vi "GAIN.vi"(0 "SR850 GPIB In":refnum<visa-resource-name>, 1 "Max. Hassasiyet":dbl=15.0, 2 "Auto Gain (False)":bool, 7 "Enum":enum16{"X", "Y"}(ring), 9 "Min. Hassasiyet":u16(ring) items=["100 nV", "200 nV", "500 nV", "1 uV", "2 uV", "5 uV", "10 uV", "20 uV", "50 uV", "100 uV", "200 uV", "500 uV", "1 mV"], 11 "error in":errorcluster, 13 "choose":dbl) -> (4 "SR850 GPIB Out":refnum<visa-resource-name>, 12 "y":dbl, 15 "error out":errorcluster)   [LabVIEW 2014]
uses:
  show_sensitivity.vi
panel:
  out "output":dbl
  out "abs(x)":dbl
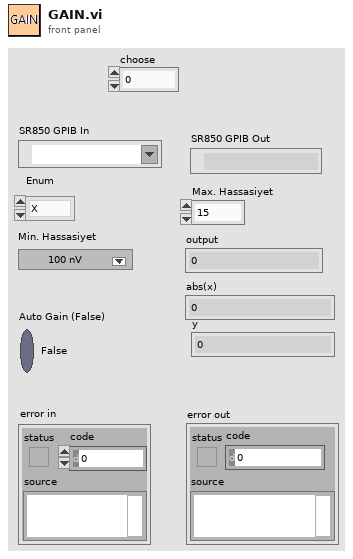
[diagram p1: front panel]
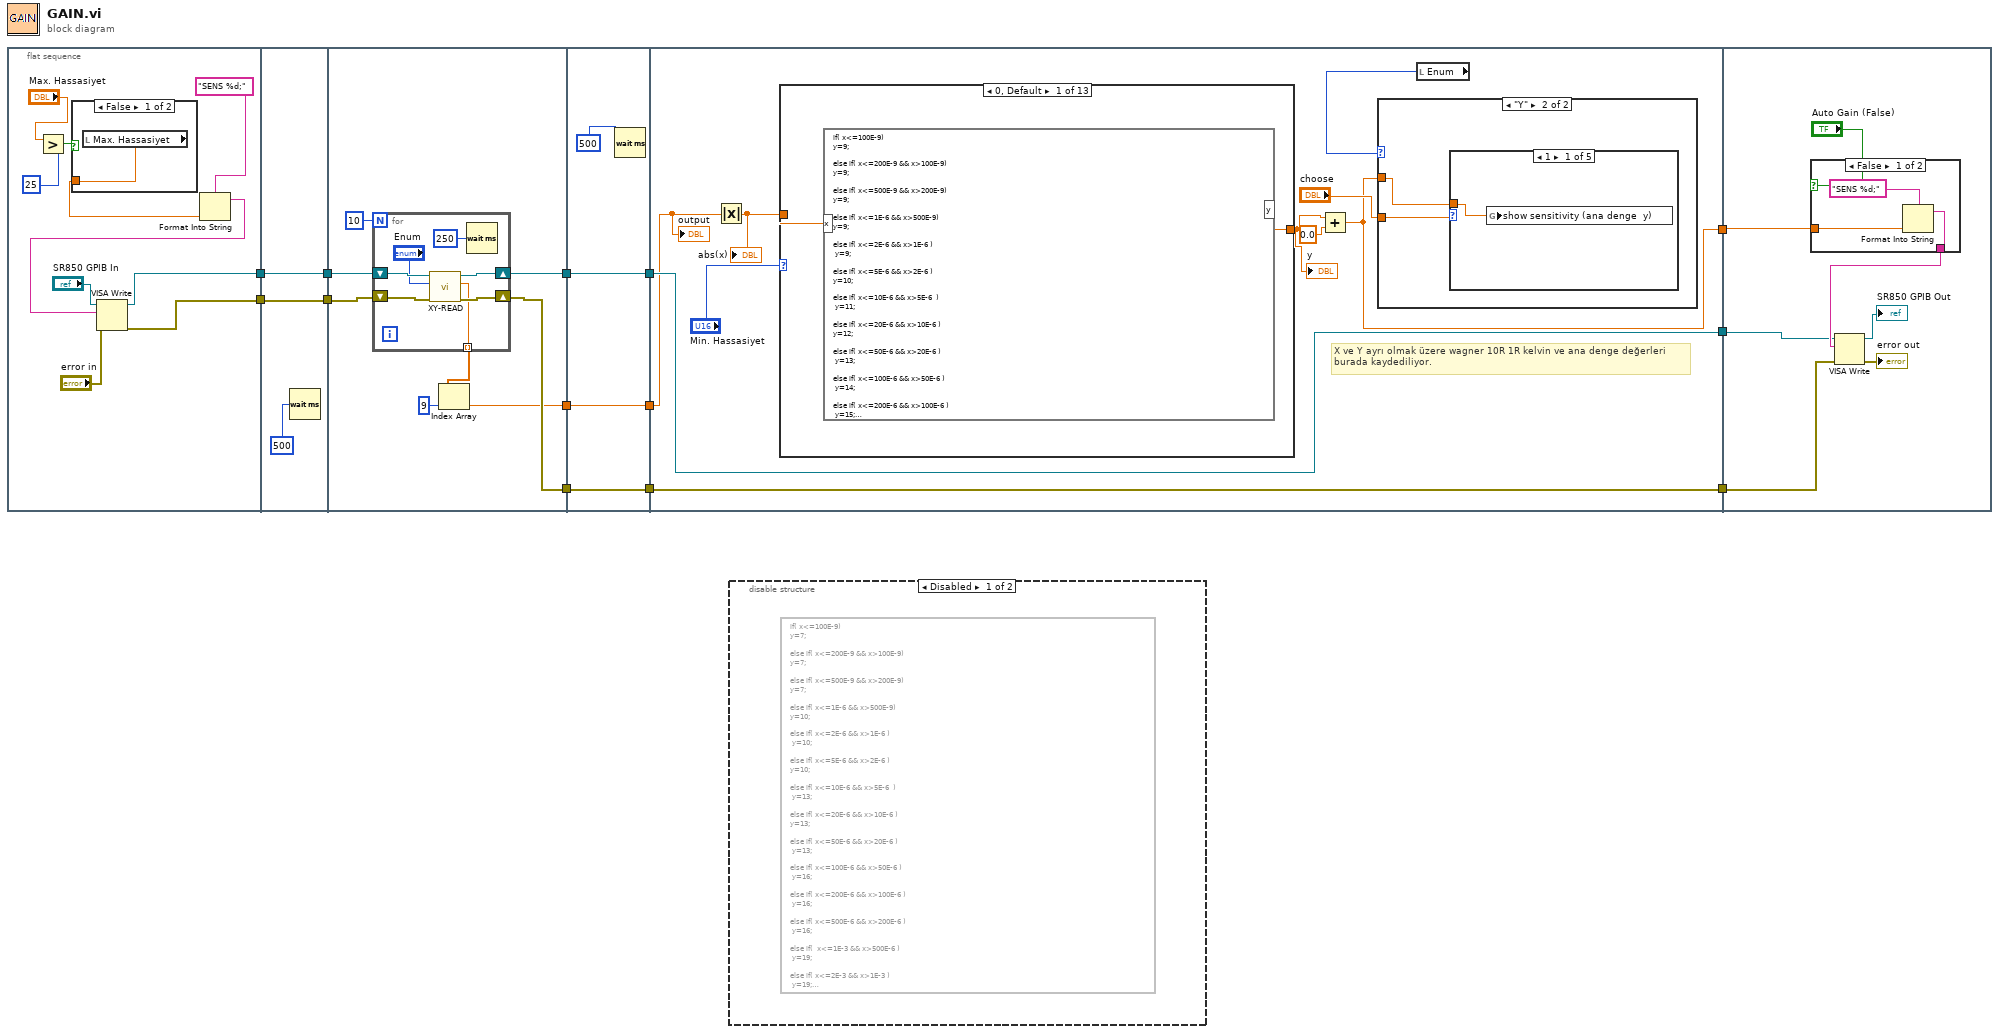
[diagram p0: block diagram]
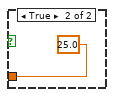
[diagram p3: hidden frame]
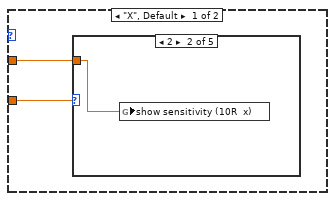
[diagram p4: hidden frame]
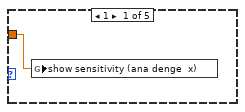
[diagram p5: hidden frame]
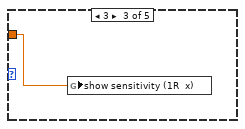
[diagram p6: hidden frame]
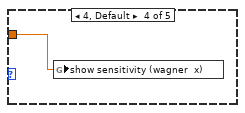
[diagram p7: hidden frame]
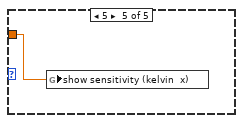
[diagram p8: hidden frame]
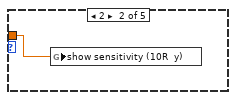
[diagram p9: hidden frame]
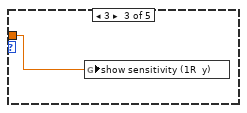
[diagram p10: hidden frame]
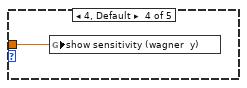
[diagram p11: hidden frame]
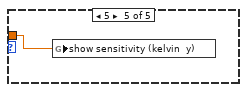
[diagram p12: hidden frame]
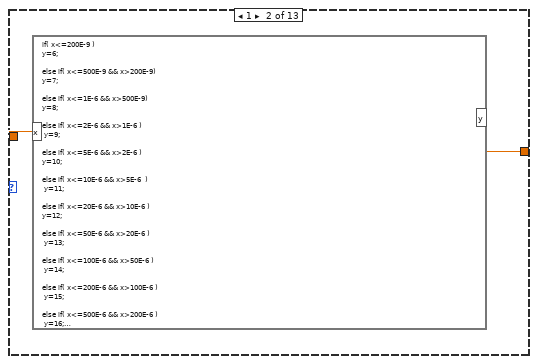
[diagram p13: hidden frame]
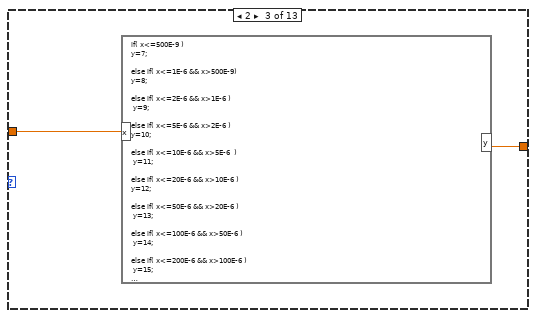
[diagram p14: hidden frame]
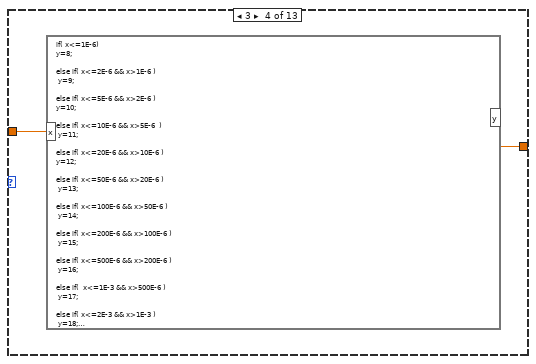
[diagram p15: hidden frame]
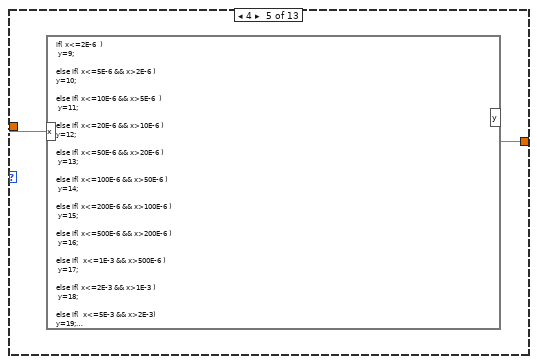
[diagram p16: hidden frame]
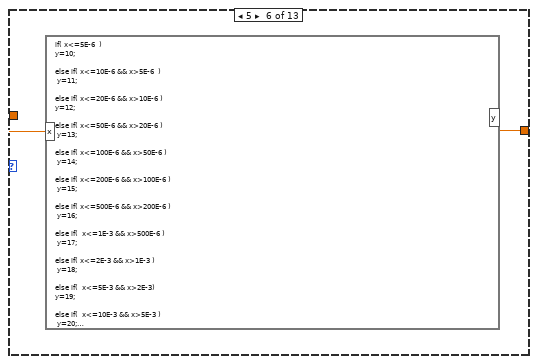
[diagram p17: hidden frame]
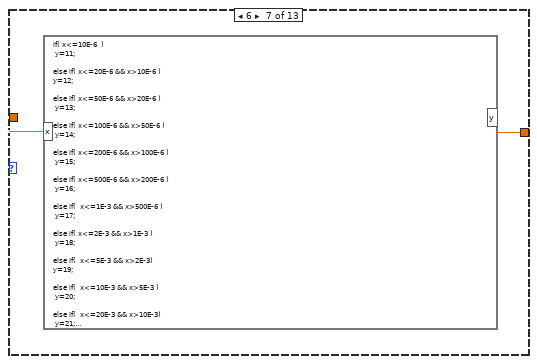
[diagram p18: hidden frame]
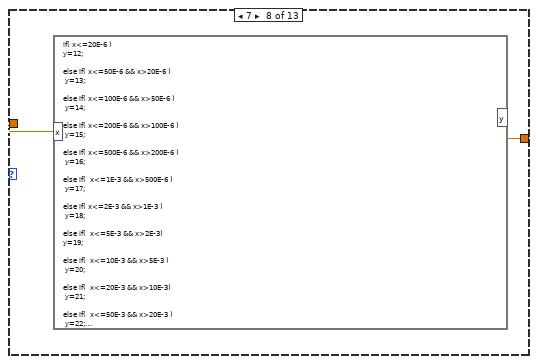
[diagram p19: hidden frame]
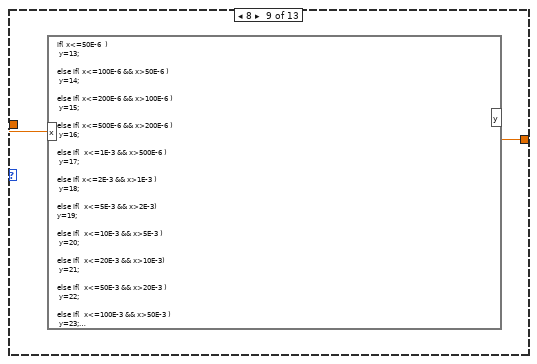
[diagram p20: hidden frame]
diagram:
  n1 = flat-sequence {
    tunnel: [w21] -> w10
    tunnel: [w18] -> w8
    tunnel: w10 -> [w28]
    tunnel: [w28] -> w9
    tunnel: w8 -> [w27]
    tunnel: [w27] -> w7
    tunnel: w9 -> [w36]
    tunnel: w7 -> [w35]
    tunnel: [w34] -> w6
    tunnel: [w33] -> w4
    tunnel: [w29] -> w2
    tunnel: w6 -> [w47]
    tunnel: [w47] -> w5
    tunnel: w4 -> [w46]
    tunnel: [w46] -> w3
    tunnel: w2 -> [w45]
    tunnel: [w45] -> w1
    tunnel: [w56] -> w13
    tunnel: w5 -> [w56]
    tunnel: [w55] -> w12
    tunnel: w3 -> [w55]
    tunnel: w1 -> [w53]
    tunnel: [w48] -> w11
    tunnel: w13 -> [w99]
    tunnel: w12 -> [w98]
    tunnel: w11 -> [w100]
    frame #0 {
      n2 = Greater?(x="Max. Hassasiyet", y=25) -> (0:w15:bool)
      n3 = case shown="False" w15 {
        tunnel: [w24 25.0] -> w14
        frame False {
          n4 = local read "Max. Hassasiyet"() -> (w24:dbl)
        }
        frame True {
        }
      }
      n5 = Format Into String(format string="SENS %d;", w14) -> (resulting string=w19:string)  [unwired: 2 in, 1 out]
      n6 = VISA Write(VISA resource name="SR850 GPIB In", write buffer=w19, error in (no error)="error in") -> (VISA resource name out=w21:refnum<visa-resource-name>, error out=w18:errorcluster)  [unwired: 1 out]
    }
    frame #1 {
      n7 = Wait (ms)(milliseconds to wait=u32 500) -> ()  [unwired: 1 out]
    }
    frame #2 {
      n8 = for {
        N: 10 -> [_]
        shift-right: [w41] -> w34
        shift-left: w36 -> [w43]
        shift-right: [w40] -> w33
        shift-left: w35 -> [w42]
        tunnel: [w38] -> w31 mode=indexing
        n9 = call "XY-READ.vi"("Error IN"=w42, "X/Y ?"="Enum", "SR850 GPIB IN"=w43) -> ("Error OUT"=w40:errorcluster, "SR850_Reading"=w38:dbl, "SR850 GPIB OUT"=w41:refnum<visa-resource-name>)  [unwired: 6 in]
        n10 = Wait (ms)(milliseconds to wait=u32 250) -> ()  [unwired: 1 out]
      }
      n11 = Index Array(array=w31, index=9) -> (element=w29:dbl)
    }
    frame #3 {
      n12 = Wait (ms)(milliseconds to wait=u32 500) -> ()  [unwired: 1 out]
    }
    frame #4 {
      # "X ve Y ayrı olmak üzere wagner 10R 1R kelvin ve ana denge değerleri\nburada kaydediliyor."
      n13 = Absolute Value(x=w53) -> (abs(x)=w54:dbl)
      "abs(x)" <- w54
      n14 = case shown="0, Default" "Min. Hassasiyet" {
        tunnel: [w73 w75 w76 w79 w81 w83 w84 w86 w88 w90 w92 w94 w96] -> w50
        tunnel: w54 -> [w72 w74 w77 w78 w80 w82 w85 w87 w89 w91 w93 w95 w97]
        frame 0, Default {
          n15 = formula code="if( x<=100E-9) \ny=9;\n\nelse if( x<=200E-9 && x>100E-9) \ny=9;\n\nelse if( x<=500E-9 && x>200E-9) \ny=9;\n\nelse if( x<=1E-6 && x>500E-9) \ny=9;\n\nelse if( x<=2E-6 && x>1E-6 ) \n\ty=9;\n\nelse if( x<=5E-6 && x>2E-6 ) \ny=10;\n\nelse if( x<=10E-6 && x>5E-6  ) \n\ty=11;\n\nelse if( x<=20E-6 && x>10E-6 ) \ny=12;\n\nelse if( x<=50E-6 && x>20E-6 ) \n\ty=13;\n\nelse if( x<=100E-6 && x>50E-6 ) \n\ty=14;\n\nelse if( x<=200E-6 && x>100E-6 ) \n\ty=15;\n\nelse if( x<=500E-6 && x>200E-6 ) \n\ty=16;\n\nelse if(  x<=1E-3 && x>500E-6 ) \n\ty=17;\n\nelse if( x<=2E-3 && x>1E-3 ) \n\ty=18;\n\nelse if(  x<=5E-3 && x>2E-3) \ny=19;\n\nelse if(  x<=10E-3 && x>5E-3 ) \n\ty=20;\n\nelse if(  x<=20E-3 && x>10E-3) \n\ty=21;\n\nelse if(  x<=50E-3 && x>20E-3 ) \n\ty=22;\n\nelse if(  x<=100E-3 && x>50E-3 ) \n\ty=23;\n\nelse if(  x<=200E-3 && x>100E-3 ) \n\ty=24;\n\nelse if(  x<=500E-3 && x>200E-3 ) \n\ty=25;\n\nelse if(  x<=1 && x>500E-3 ) \ny=26;\n\nelse \n\ty=26;"("x"=w72) -> ("y"=w73:dbl)
        }
        frame 1 {
          n16 = formula code="if( x<=200E-9 ) \ny=6;\n\nelse if( x<=500E-9 && x>200E-9) \ny=7;\n\nelse if( x<=1E-6 && x>500E-9) \ny=8;\n\nelse if( x<=2E-6 && x>1E-6 ) \n\ty=9;\n\nelse if( x<=5E-6 && x>2E-6 ) \ny=10;\n\nelse if( x<=10E-6 && x>5E-6  ) \n\ty=11;\n\nelse if( x<=20E-6 && x>10E-6 ) \ny=12;\n\nelse if( x<=50E-6 && x>20E-6 ) \n\ty=13;\n\nelse if( x<=100E-6 && x>50E-6 ) \n\ty=14;\n\nelse if( x<=200E-6 && x>100E-6 ) \n\ty=15;\n\nelse if( x<=500E-6 && x>200E-6 ) \n\ty=16;\n\nelse if(  x<=1E-3 && x>500E-6 ) \n\ty=17;\n\nelse if( x<=2E-3 && x>1E-3 ) \n\ty=18;\n\nelse if(  x<=5E-3 && x>2E-3) \ny=19;\n\nelse if(  x<=10E-3 && x>5E-3 ) \n\ty=20;\n\nelse if(  x<=20E-3 && x>10E-3) \n\ty=21;\n\nelse if(  x<=50E-3 && x>20E-3 ) \n\ty=22;\n\nelse if(  x<=100E-3 && x>50E-3 ) \n\ty=23;\n\nelse if(  x<=200E-3 && x>100E-3 ) \n\ty=24;\n\nelse if(  x<=500E-3 && x>200E-3 ) \n\ty=25;\n\nelse if(  x<=1 && x>500E-3 ) \ny=26;\n\nelse \n\ty=26;"("x"=w74) -> ("y"=w75:dbl)
        }
        frame 2 {
          n17 = formula code="if( x<=500E-9 ) \ny=7;\n\nelse if( x<=1E-6 && x>500E-9) \ny=8;\n\nelse if( x<=2E-6 && x>1E-6 ) \n\ty=9;\n\nelse if( x<=5E-6 && x>2E-6 ) \ny=10;\n\nelse if( x<=10E-6 && x>5E-6  ) \n\ty=11;\n\nelse if( x<=20E-6 && x>10E-6 ) \ny=12;\n\nelse if( x<=50E-6 && x>20E-6 ) \n\ty=13;\n\nelse if( x<=100E-6 && x>50E-6 ) \n\ty=14;\n\nelse if( x<=200E-6 && x>100E-6 ) \n\ty=15;\n\nelse if( x<=500E-6 && x>200E-6 ) \n\ty=16;\n\nelse if(  x<=1E-3 && x>500E-6 ) \n\ty=17;\n\nelse if( x<=2E-3 && x>1E-3 ) \n\ty=18;\n\nelse if(  x<=5E-3 && x>2E-3) \ny=19;\n\nelse if(  x<=10E-3 && x>5E-3 ) \n\ty=20;\n\nelse if(  x<=20E-3 && x>10E-3) \n\ty=21;\n\nelse if(  x<=50E-3 && x>20E-3 ) \n\ty=22;\n\nelse if(  x<=100E-3 && x>50E-3 ) \n\ty=23;\n\nelse if(  x<=200E-3 && x>100E-3 ) \n\ty=24;\n\nelse if(  x<=500E-3 && x>200E-3 ) \n\ty=25;\n\nelse if(  x<=1 && x>500E-3 ) \ny=26;\n\nelse \n\ty=26;"("x"=w77) -> ("y"=w76:dbl)
        }
        frame 3 {
          n18 = formula code="if( x<=1E-6) \ny=8;\n\nelse if( x<=2E-6 && x>1E-6 ) \n\ty=9;\n\nelse if( x<=5E-6 && x>2E-6 ) \ny=10;\n\nelse if( x<=10E-6 && x>5E-6  ) \n\ty=11;\n\nelse if( x<=20E-6 && x>10E-6 ) \ny=12;\n\nelse if( x<=50E-6 && x>20E-6 ) \n\ty=13;\n\nelse if( x<=100E-6 && x>50E-6 ) \n\ty=14;\n\nelse if( x<=200E-6 && x>100E-6 ) \n\ty=15;\n\nelse if( x<=500E-6 && x>200E-6 ) \n\ty=16;\n\nelse if(  x<=1E-3 && x>500E-6 ) \n\ty=17;\n\nelse if( x<=2E-3 && x>1E-3 ) \n\ty=18;\n\nelse if(  x<=5E-3 && x>2E-3) \ny=19;\n\nelse if(  x<=10E-3 && x>5E-3 ) \n\ty=20;\n\nelse if(  x<=20E-3 && x>10E-3) \n\ty=21;\n\nelse if(  x<=50E-3 && x>20E-3 ) \n\ty=22;\n\nelse if(  x<=100E-3 && x>50E-3 ) \n\ty=23;\n\nelse if(  x<=200E-3 && x>100E-3 ) \n\ty=24;\n\nelse if(  x<=500E-3 && x>200E-3 ) \n\ty=25;\n\nelse if(  x<=1 && x>500E-3 ) \ny=26;\n\nelse \n\ty=26;"("x"=w78) -> ("y"=w79:dbl)
        }
        frame 4 {
          n19 = formula code="if( x<=2E-6  ) \n\ty=9;\n\nelse if( x<=5E-6 && x>2E-6 ) \ny=10;\n\nelse if( x<=10E-6 && x>5E-6  ) \n\ty=11;\n\nelse if( x<=20E-6 && x>10E-6 ) \ny=12;\n\nelse if( x<=50E-6 && x>20E-6 ) \n\ty=13;\n\nelse if( x<=100E-6 && x>50E-6 ) \n\ty=14;\n\nelse if( x<=200E-6 && x>100E-6 ) \n\ty=15;\n\nelse if( x<=500E-6 && x>200E-6 ) \n\ty=16;\n\nelse if(  x<=1E-3 && x>500E-6 ) \n\ty=17;\n\nelse if( x<=2E-3 && x>1E-3 ) \n\ty=18;\n\nelse if(  x<=5E-3 && x>2E-3) \ny=19;\n\nelse if(  x<=10E-3 && x>5E-3 ) \n\ty=20;\n\nelse if(  x<=20E-3 && x>10E-3) \n\ty=21;\n\nelse if(  x<=50E-3 && x>20E-3 ) \n\ty=22;\n\nelse if(  x<=100E-3 && x>50E-3 ) \n\ty=23;\n\nelse if(  x<=200E-3 && x>100E-3 ) \n\ty=24;\n\nelse if(  x<=500E-3 && x>200E-3 ) \n\ty=25;\n\nelse if(  x<=1 && x>500E-3 ) \ny=26;\n\nelse \n\ty=26;"("x"=w80) -> ("y"=w81:dbl)
        }
        frame 5 {
          n20 = formula code="if( x<=5E-6  ) \ny=10;\n\nelse if( x<=10E-6 && x>5E-6  ) \n\ty=11;\n\nelse if( x<=20E-6 && x>10E-6 ) \ny=12;\n\nelse if( x<=50E-6 && x>20E-6 ) \n\ty=13;\n\nelse if( x<=100E-6 && x>50E-6 ) \n\ty=14;\n\nelse if( x<=200E-6 && x>100E-6 ) \n\ty=15;\n\nelse if( x<=500E-6 && x>200E-6 ) \n\ty=16;\n\nelse if(  x<=1E-3 && x>500E-6 ) \n\ty=17;\n\nelse if( x<=2E-3 && x>1E-3 ) \n\ty=18;\n\nelse if(  x<=5E-3 && x>2E-3) \ny=19;\n\nelse if(  x<=10E-3 && x>5E-3 ) \n\ty=20;\n\nelse if(  x<=20E-3 && x>10E-3) \n\ty=21;\n\nelse if(  x<=50E-3 && x>20E-3 ) \n\ty=22;\n\nelse if(  x<=100E-3 && x>50E-3 ) \n\ty=23;\n\nelse if(  x<=200E-3 && x>100E-3 ) \n\ty=24;\n\nelse if(  x<=500E-3 && x>200E-3 ) \n\ty=25;\n\nelse if(  x<=1 && x>500E-3 ) \ny=26;\n\nelse \n\ty=26;"("x"=w82) -> ("y"=w83:dbl)
        }
        frame 6 {
          n21 = formula code="if( x<=10E-6  ) \n\ty=11;\n\nelse if( x<=20E-6 && x>10E-6 ) \ny=12;\n\nelse if( x<=50E-6 && x>20E-6 ) \n\ty=13;\n\nelse if( x<=100E-6 && x>50E-6 ) \n\ty=14;\n\nelse if( x<=200E-6 && x>100E-6 ) \n\ty=15;\n\nelse if( x<=500E-6 && x>200E-6 ) \n\ty=16;\n\nelse if(  x<=1E-3 && x>500E-6 ) \n\ty=17;\n\nelse if( x<=2E-3 && x>1E-3 ) \n\ty=18;\n\nelse if(  x<=5E-3 && x>2E-3) \ny=19;\n\nelse if(  x<=10E-3 && x>5E-3 ) \n\ty=20;\n\nelse if(  x<=20E-3 && x>10E-3) \n\ty=21;\n\nelse if(  x<=50E-3 && x>20E-3 ) \n\ty=22;\n\nelse if(  x<=100E-3 && x>50E-3 ) \n\ty=23;\n\nelse if(  x<=200E-3 && x>100E-3 ) \n\ty=24;\n\nelse if(  x<=500E-3 && x>200E-3 ) \n\ty=25;\n\nelse if(  x<=1 && x>500E-3 ) \ny=26;\n\nelse \n\ty=26;"("x"=w85) -> ("y"=w84:dbl)
        }
        frame 7 {
          n22 = formula code="if( x<=20E-6 ) \ny=12;\n\nelse if( x<=50E-6 && x>20E-6 ) \n\ty=13;\n\nelse if( x<=100E-6 && x>50E-6 ) \n\ty=14;\n\nelse if( x<=200E-6 && x>100E-6 ) \n\ty=15;\n\nelse if( x<=500E-6 && x>200E-6 ) \n\ty=16;\n\nelse if(  x<=1E-3 && x>500E-6 ) \n\ty=17;\n\nelse if( x<=2E-3 && x>1E-3 ) \n\ty=18;\n\nelse if(  x<=5E-3 && x>2E-3) \ny=19;\n\nelse if(  x<=10E-3 && x>5E-3 ) \n\ty=20;\n\nelse if(  x<=20E-3 && x>10E-3) \n\ty=21;\n\nelse if(  x<=50E-3 && x>20E-3 ) \n\ty=22;\n\nelse if(  x<=100E-3 && x>50E-3 ) \n\ty=23;\n\nelse if(  x<=200E-3 && x>100E-3 ) \n\ty=24;\n\nelse if(  x<=500E-3 && x>200E-3 ) \n\ty=25;\n\nelse if(  x<=1 && x>500E-3 ) \ny=26;\n\nelse \n\ty=26;"("x"=w87) -> ("y"=w86:dbl)
        }
        frame 8 {
          n23 = formula code="if( x<=50E-6  ) \n\ty=13;\n\nelse if( x<=100E-6 && x>50E-6 ) \n\ty=14;\n\nelse if( x<=200E-6 && x>100E-6 ) \n\ty=15;\n\nelse if( x<=500E-6 && x>200E-6 ) \n\ty=16;\n\nelse if(  x<=1E-3 && x>500E-6 ) \n\ty=17;\n\nelse if( x<=2E-3 && x>1E-3 ) \n\ty=18;\n\nelse if(  x<=5E-3 && x>2E-3) \ny=19;\n\nelse if(  x<=10E-3 && x>5E-3 ) \n\ty=20;\n\nelse if(  x<=20E-3 && x>10E-3) \n\ty=21;\n\nelse if(  x<=50E-3 && x>20E-3 ) \n\ty=22;\n\nelse if(  x<=100E-3 && x>50E-3 ) \n\ty=23;\n\nelse if(  x<=200E-3 && x>100E-3 ) \n\ty=24;\n\nelse if(  x<=500E-3 && x>200E-3 ) \n\ty=25;\n\nelse if(  x<=1 && x>500E-3 ) \ny=26;\n\nelse \n\ty=26;"("x"=w89) -> ("y"=w88:dbl)
        }
        frame 9 {
          n24 = formula code="if( x<=100E-6 ) \n\ty=14;\n\nelse if( x<=200E-6 && x>100E-6 ) \n\ty=15;\n\nelse if( x<=500E-6 && x>200E-6 ) \n\ty=16;\n\nelse if(  x<=1E-3 && x>500E-6 ) \n\ty=17;\n\nelse if( x<=2E-3 && x>1E-3 ) \n\ty=18;\n\nelse if(  x<=5E-3 && x>2E-3) \ny=19;\n\nelse if(  x<=10E-3 && x>5E-3 ) \n\ty=20;\n\nelse if(  x<=20E-3 && x>10E-3) \n\ty=21;\n\nelse if(  x<=50E-3 && x>20E-3 ) \n\ty=22;\n\nelse if(  x<=100E-3 && x>50E-3 ) \n\ty=23;\n\nelse if(  x<=200E-3 && x>100E-3 ) \n\ty=24;\n\nelse if(  x<=500E-3 && x>200E-3 ) \n\ty=25;\n\nelse if(  x<=1 && x>500E-3 ) \ny=26;\n\nelse \n\ty=26;"("x"=w91) -> ("y"=w90:dbl)
        }
        frame 10 {
          n25 = formula code="if( x<=200E-6 ) \n\ty=15;\n\nelse if( x<=500E-6 && x>200E-6 ) \n\ty=16;\n\nelse if(  x<=1E-3 && x>500E-6 ) \n\ty=17;\n\nelse if( x<=2E-3 && x>1E-3 ) \n\ty=18;\n\nelse if(  x<=5E-3 && x>2E-3) \ny=19;\n\nelse if(  x<=10E-3 && x>5E-3 ) \n\ty=20;\n\nelse if(  x<=20E-3 && x>10E-3) \n\ty=21;\n\nelse if(  x<=50E-3 && x>20E-3 ) \n\ty=22;\n\nelse if(  x<=100E-3 && x>50E-3 ) \n\ty=23;\n\nelse if(  x<=200E-3 && x>100E-3 ) \n\ty=24;\n\nelse if(  x<=500E-3 && x>200E-3 ) \n\ty=25;\n\nelse if(  x<=1 && x>500E-3 ) \ny=26;\n\nelse \n\ty=26;"("x"=w93) -> ("y"=w92:dbl)
        }
        frame 11 {
          n26 = formula code="if( x<=500E-6 ) \n\ty=16;\n\nelse if(  x<=1E-3 && x>500E-6 ) \n\ty=17;\n\nelse if( x<=2E-3 && x>1E-3 ) \n\ty=18;\n\nelse if(  x<=5E-3 && x>2E-3) \ny=19;\n\nelse if(  x<=10E-3 && x>5E-3 ) \n\ty=20;\n\nelse if(  x<=20E-3 && x>10E-3) \n\ty=21;\n\nelse if(  x<=50E-3 && x>20E-3 ) \n\ty=22;\n\nelse if(  x<=100E-3 && x>50E-3 ) \n\ty=23;\n\nelse if(  x<=200E-3 && x>100E-3 ) \n\ty=24;\n\nelse if(  x<=500E-3 && x>200E-3 ) \n\ty=25;\n\nelse if(  x<=1 && x>500E-3 ) \ny=26;\n\nelse \n\ty=26;"("x"=w95) -> ("y"=w94:dbl)
        }
        frame 12 {
          n27 = formula code="if(  x<=1E-3  ) \n\ty=17;\n\nelse if( x<=2E-3 && x>1E-3 ) \n\ty=18;\n\nelse if(  x<=5E-3 && x>2E-3) \ny=19;\n\nelse if(  x<=10E-3 && x>5E-3 ) \n\ty=20;\n\nelse if(  x<=20E-3 && x>10E-3) \n\ty=21;\n\nelse if(  x<=50E-3 && x>20E-3 ) \n\ty=22;\n\nelse if(  x<=100E-3 && x>50E-3 ) \n\ty=23;\n\nelse if(  x<=200E-3 && x>100E-3 ) \n\ty=24;\n\nelse if(  x<=500E-3 && x>200E-3 ) \n\ty=25;\n\nelse if(  x<=1 && x>500E-3 ) \ny=26;\n\nelse \n\ty=26;"("x"=w97) -> ("y"=w96:dbl)
        }
      }
      "y" <- w50
      n28 = Add(x=w50, y=0.0) -> (x+y=w48:dbl)
      n29 = local read "Enum"() -> (w52:enum16{"X", "Y"})
      n30 = case shown="\"Y\"" w52 {
        tunnel: w48 -> [w58 w65]
        tunnel: "choose" -> [w59 w66]
        frame "X", Default {
          n31 = case shown="2" w59 {
            tunnel: w58 -> [w60 w61 w62 w63 w64]
            frame 1 {
              n32 = global write "show_sensitivity.vi" "show sensitivity (ana denge  x)"(w60) -> ()
            }
            frame 2 {
              n33 = global write "show_sensitivity.vi" "show sensitivity (10R  x)"(w61) -> ()
            }
            frame 3 {
              n34 = global write "show_sensitivity.vi" "show sensitivity (1R  x)"(w62) -> ()
            }
            frame 4, Default {
              n35 = global write "show_sensitivity.vi" "show sensitivity (wagner  x)"(w63) -> ()
            }
            frame 5 {
              n36 = global write "show_sensitivity.vi" "show sensitivity (kelvin  x)"(w64) -> ()
            }
          }
        }
        frame "Y" {
          n37 = case shown="1" w66 {
            tunnel: w65 -> [w67 w68 w69 w70 w71]
            frame 1 {
              n38 = global write "show_sensitivity.vi" "show sensitivity (ana denge  y)"(w67) -> ()
            }
            frame 2 {
              n39 = global write "show_sensitivity.vi" "show sensitivity (10R  y)"(w68) -> ()
            }
            frame 3 {
              n40 = global write "show_sensitivity.vi" "show sensitivity (1R  y)"(w69) -> ()
            }
            frame 4, Default {
              n41 = global write "show_sensitivity.vi" "show sensitivity (wagner  y)"(w70) -> ()
            }
            frame 5 {
              n42 = global write "show_sensitivity.vi" "show sensitivity (kelvin  y)"(w71) -> ()
            }
          }
        }
      }
      "output" <- w53
    }
    frame #5 {
      n43 = case shown="False" "Auto Gain (False)" {
        tunnel: [w106 "AGAN;" ("true string")] -> w101
        tunnel: w100 -> [w105 _]
        frame False {
          n44 = Format Into String(format string="SENS %d;", w105) -> (resulting string=w106:string)  [unwired: 2 in, 1 out]
        }
        frame True {
        }
      }
      n45 = VISA Write(VISA resource name=w99, write buffer=w101, error in (no error)=w98) -> (VISA resource name out=→"SR850 GPIB Out":refnum<visa-resource-name>, error out=→"error out":errorcluster)  [unwired: 1 out]
    }
  }
  n46 = disable-structure shown="Disabled" {
    frame Disabled {
      n47 = formula code="if( x<=100E-9) \ny=7;\n\nelse if( x<=200E-9 && x>100E-9) \ny=7;\n\nelse if( x<=500E-9 && x>200E-9) \ny=7;\n\nelse if( x<=1E-6 && x>500E-9) \ny=10;\n\nelse if( x<=2E-6 && x>1E-6 ) \n\ty=10;\n\nelse if( x<=5E-6 && x>2E-6 ) \ny=10;\n\nelse if( x<=10E-6 && x>5E-6  ) \n\ty=13;\n\nelse if( x<=20E-6 && x>10E-6 ) \ny=13;\n\nelse if( x<=50E-6 && x>20E-6 ) \n\ty=13;\n\nelse if( x<=100E-6 && x>50E-6 ) \n\ty=16;\n\nelse if( x<=200E-6 && x>100E-6 ) \n\ty=16;\n\nelse if( x<=500E-6 && x>200E-6 ) \n\ty=16;\n\nelse if(  x<=1E-3 && x>500E-6 ) \n\ty=19;\n\nelse if( x<=2E-3 && x>1E-3 ) \n\ty=19;\n\nelse if(  x<=5E-3 && x>2E-3) \ny=19;\n\nelse if(  x<=10E-3 && x>5E-3 ) \n\ty=22;\n\nelse if(  x<=20E-3 && x>10E-3) \n\ty=22;\n\nelse if(  x<=50E-3 && x>20E-3 ) \n\ty=22;\n\nelse if(  x<=100E-3 && x>50E-3 ) \n\ty=25;\n\nelse if(  x<=200E-3 && x>100E-3 ) \n\ty=25;\n\nelse if(  x<=500E-3 && x>200E-3 ) \n\ty=25;\n\nelse if(  x<=1 && x>500E-3 ) \ny=26;\n\nelse \n\ty=26;"() -> ()
    }
    frame Enabled {
    }
  }
